vi "Set State by Index.vi"(8 "error in (no error)":errorcluster, 9 "Enum":T1, 10 "index":i32, 11 "Example App Properties in":refnum<class "Example App Properties.lvclass">) -> (0 "error out":errorcluster, 3 "Example App Properties out":refnum<class "Example App Properties.lvclass">)   [LabVIEW 2015, in "Example Application.lvlib" / "Example App Properties.lvclass"]
uses:
  Example App Properties.lvclass
  DUT State -- Enum.ctl
  Example App Properties.lvclass/Example App Properties.ctl
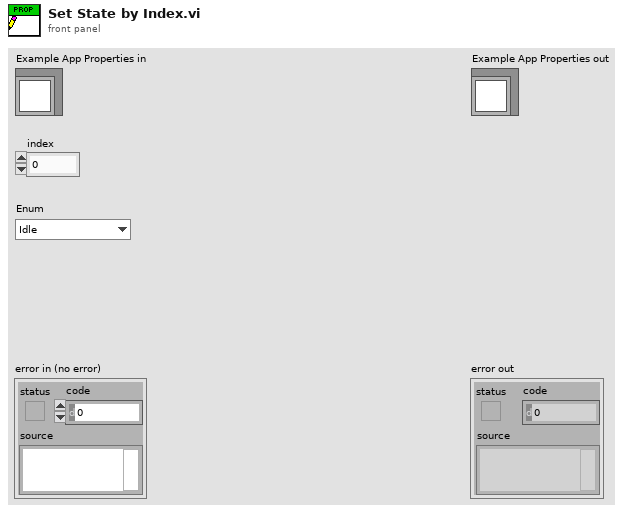
[diagram p1: front panel]
types:
  T1 = typedef "Example Application.lvlib/Example App Properties.lvclass/DUT State -- Enum.ctl" = enum16{"Idle", "Testing", "Passed", "Failed"}
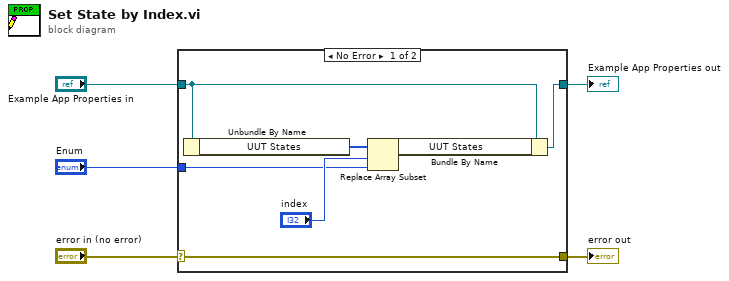
[diagram p0: block diagram]
diagram:
  n1 = case shown="No Error" "error in (no error)" {
    selector: "error in (no error)" -> [w12 w13]
    tunnel: [w12 w13] -> w4
    tunnel: [w11 w14] -> w2
    tunnel: "Example App Properties in" -> [w10 w14]
    tunnel: "Enum" -> [w6 _]
    frame No Error {
      n2 = Unbundle By Name(w10) -> ("UUT States"=w9:T1[])
      n3 = Replace Array Subset(array=w9, new element=w6, index="index") -> (w8:T1[])
      n4 = Bundle By Name(cluster=w10, "UUT States"=w8) -> (w11:refnum<class "Example App Properties.lvclass">)
    }
    frame Error {
    }
  }
  "error out" <- w4
  "Example App Properties out" <- w2
